vi "Test Fichiers.vi"() -> ()   [LabVIEW 2026]
uses:
  7cfcc2c8-74b8-44a5-aa8a-30382eebebdc.vi
  7cfcc2c8-74b8-44a5-aa8a-30382eebebdc.vi/659df739-fa42-474c-bf03-f9ba45f35773.vi
  <userlib>/LV-TOML/lib/Write TOML File (LV).vi
  <userlib>/LV-TOML/lib/Parse TOML String.vi
  <userlib>/LV-TOML/lib/TOML to LabVIEW.vi
  <userlib>/LV-TOML/lib/LV-TOML.lvlib
panel:
  out "Chaine de caractère":string
  out "Nbre":i32
  in  "Data":T1={"Nbre"=0, "Chaine de caractère"="", "Tableau"=[], "Cluster"={"1"=TRUE, "2"=TRUE, "3"=TRUE}}
  out "error out":errorcluster caption="sortie d'erreur"
  in  "error in (no error)":errorcluster caption="entrée d'erreur (pas d'erreur)"
  out "file or folder exists?":bool caption="le fichier ou dossier existe ?"
  in  "Énum":T2(ring)
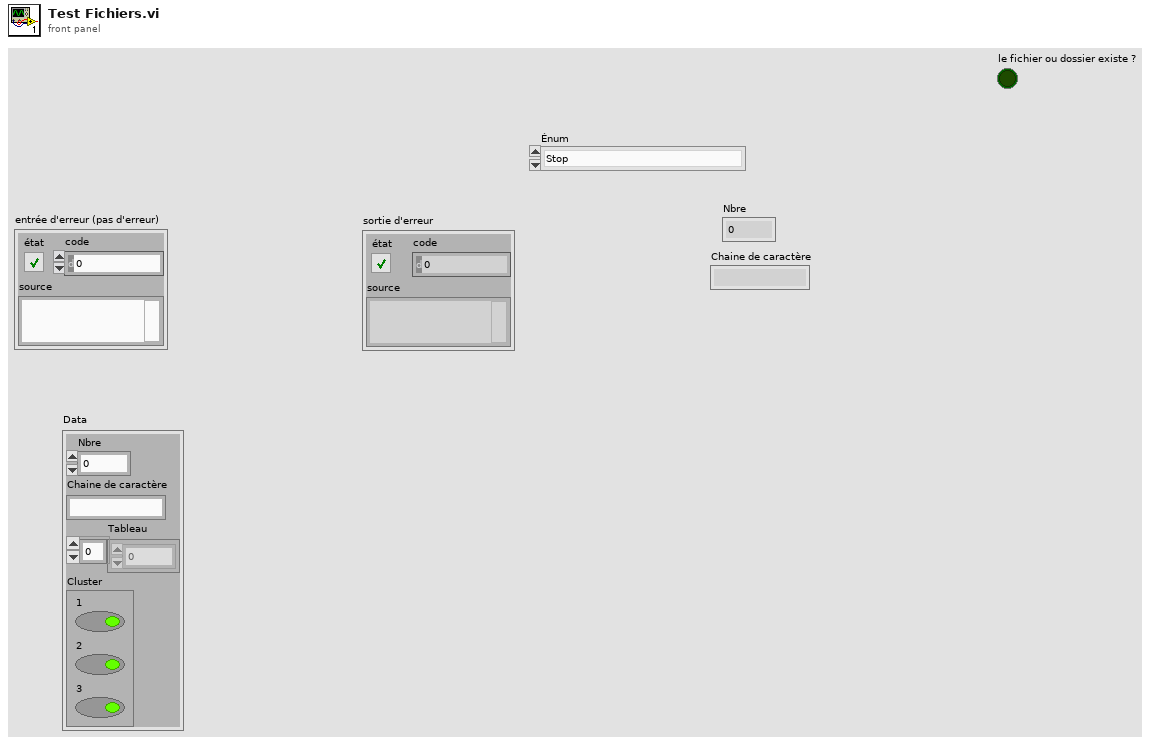
[diagram p1: front panel]
types:
  T1 = cluster{"Nbre":i32, "Chaine de caractère":string, "Tableau":i16[], "Cluster":cluster{"1":bool, "2":bool, "3":bool}}
  T2 = enum16{"Stop", "Enregitrer Data", "Lecture Data", "Initialiser", "Erreur"}
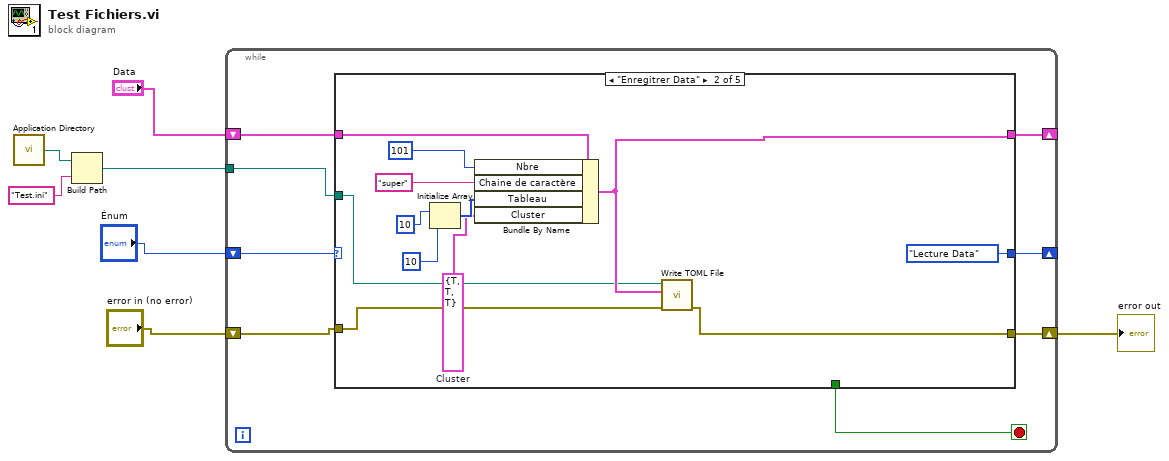
[diagram p0: block diagram]
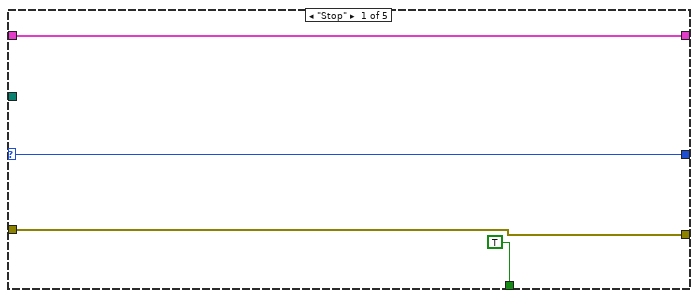
[diagram p2: hidden frame]
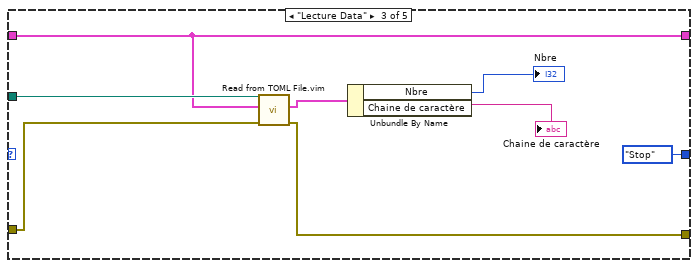
[diagram p3: hidden frame]
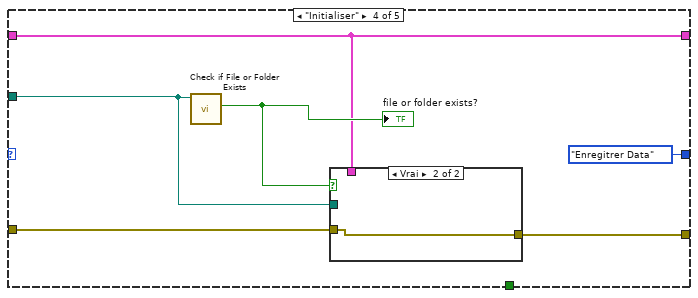
[diagram p4: hidden frame]
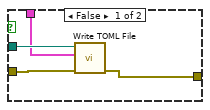
[diagram p5: hidden frame]
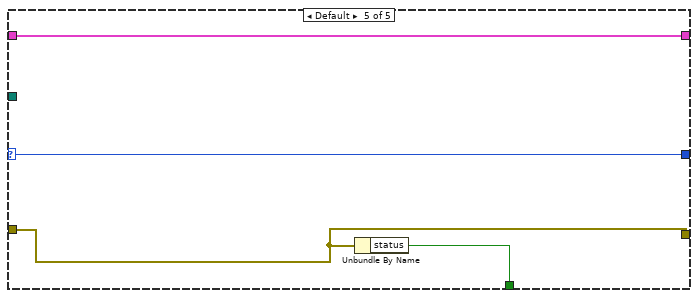
[diagram p6: hidden frame]
diagram:
  n1 = call <vilib>:"Application Directory.vi"() -> ("Application Directory"=w3:path)
  n2 = Build Path(base path=w3, name or relative path="Test.ini") -> (appended path=w1:path)
  n3 = while {
    shift-right: [w14] -> _
    shift-left: "Énum" -> [w15]
    shift-right: [w11] -> w5
    shift-left: "error in (no error)" -> [w12]
    shift-right: [w10] -> _
    shift-left: "Data" -> [w9]
    tunnel: w1 -> [w8]
    stop <- w13 stop-if-true
    n4 = case shown="\"Enregitrer Data\"" w15 {
      selector: w15 -> [w19 _ _ _ w54]
      tunnel: [w19 T2."Lecture Data" ("Énum") T2."Stop" ("Énum") T2."Enregitrer Data" ("Énum") w54] -> w14
      tunnel: [TRUE _ _ _ w53] -> w13
      tunnel: w12 -> [w17 w30 w39 w45 w52]
      tunnel: [w17 w29 w38 w44 w52] -> w11
      tunnel: [w16 w28 w36 w42 w51] -> w10
      tunnel: w9 -> [w16 w31 w36 w42 w51]
      tunnel: w8 -> [_ w27 w37 w40 _]
      frame "Stop" {
      }
      frame "Enregitrer Data" {
        w20 = cluster{"1":bool, "2":bool, "3":bool} {"1"=TRUE, "2"=TRUE, "3"=TRUE}  # Cluster
        n5 = Initialize Array(i16 10 ("élément"), 10 ("taille de la dimension")) -> (w21:i16[])
        n6 = Bundle By Name(cluster=w31, "Nbre"=101, "Chaine de caractère"="super", "Tableau"=w21, "Cluster"=w20) -> (w28:T1)
        n7 = call-poly <userlib>:"Write TOML File.vi"("error in (no error)"=w30, "Value"=w28, "file path (use dialog)"=w27) -> ("error out"=w29:errorcluster)  [unwired: 8 in]
      }
      frame "Lecture Data" {
        n8 = call "Read from TOML File.vim"("error in (no error)"=w39, "Default Value"=w36, "file path (use dialog)"=w37) -> ("error out"=w38:errorcluster, "Value"=w35:T1)  [unwired: 6 in, 1 out]
        n9 = Unbundle By Name(w35) -> ("Nbre"=→"Nbre":i32, "Chaine de caractère"=→"Chaine de caractère":string)
      }
      frame "Initialiser" {
        n10 = call <vilib>:"Check if File or Folder Exists.vi"("path"=w40) -> ("file or folder exists?"=w43:bool)  [unwired: 8 in, 2 out]
        "file or folder exists?" <- w43
        n11 = case shown="Vrai" w43 {
          tunnel: w45 -> [w49 w50]
          tunnel: [w48 w50] -> w44
          tunnel: w40 -> [w47 _]
          tunnel: w42 -> [w46 _]
          frame False {
            n12 = call-poly <userlib>:"Write TOML File.vi"("error in (no error)"=w49, "Value"=w46, "file path (use dialog)"=w47) -> ("error out"=w48:errorcluster)  [unwired: 8 in]
          }
          frame True {
          }
        }
      }
      frame Default {
        n13 = Unbundle By Name(w52) -> ("status"=w53:bool)
      }
    }
  }
  "error out" <- w5
